vi "Initialize.vi"(6 "timeout in ms":i32=2000, 7 "Engine Configuration":refnum<class "engine configuration.lvclass">, 8 "error in":errorcluster, 9 "module Configurations":refnum<class "TBM module configuration.lvclass">[](array[class]), 10 "modules":refnum<class "TBM module execution interface.lvclass">[](array[class]), 11 "Engine Runtime Interface in":refnum<class "Engine Runtime Interface.lvclass">) -> (0 "error out":errorcluster, 3 "Engine Runtime Interface out":refnum<class "Engine Runtime Interface.lvclass">)   [LabVIEW 2013, in "Engine Runtime Interface.lvclass"]
uses:
  Engine Runtime Interface.lvclass
  <vilib>/NI/Tag Bus Module Framework/module configuration/TBM module configuration.lvclass
  <vilib>/NI/Tag Bus Module Framework/runtime/TBM module execution interface.lvclass
  Engine Configuration/engine configuration.lvclass
  <vilib>/NI/CEF/CEF_TreeControl/NISE_CEF_TreeControl.lvlib
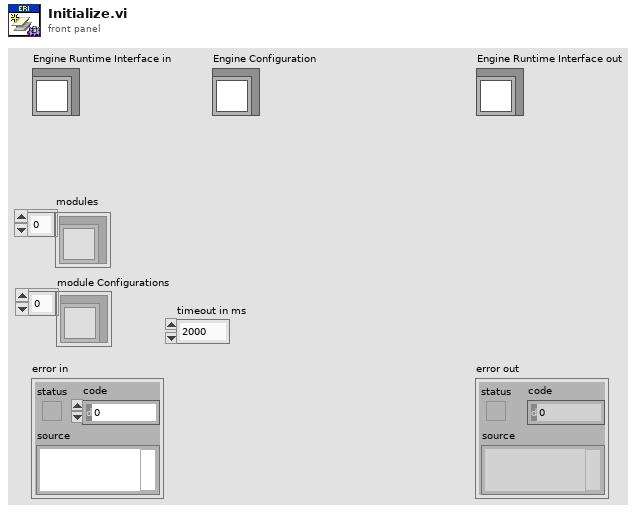
[diagram p1: front panel]
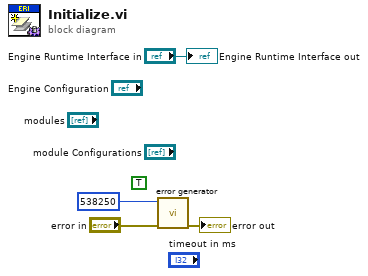
[diagram p0: block diagram]
diagram:
  (unwired) TRUE ("show call chain? (False)")
  n1 = call <vilib>:"error generator.vi"("error in"="error in", "error code (0)"=538250) -> ("error out"=→"error out":errorcluster)  [unwired: 7 in]
  "Engine Runtime Interface out" <- "Engine Runtime Interface in"
